vi "niWLAN - OPPO - 80211abgnIQMeasurementsSettings.vi"(0 "niwlan analysis session":T6, 1 "WLAN Measurement Settings":T1={"OFDM Advanced Controls(11ag)"={"OFDM Auto Compute Acquisition Length Enabled"=0, "OFDM Maximum Symbols Used"=0, "OFDM Time Tracking Enabled"=0, "OFDM Channel Tracking Enabled"=0, "OFDM Amplitude Tracking Enabled"=1, "OFDM CFO Estimation Method"=0, "OFDM Phase Tracking Method"=0, "OFDM Header Detection Enabled"=0, "OFDM MAC FCS Check Enabled"=0, "#Avg"=10, "#Iterations"=10}, "DSSS Demod Parameters"={"DSSS Auto Compute Acquisition Length Enabled"=0, "DSSS Equalization Enabled"=0, "DSSS Header Detection Enabled"=0, "DSSS MAC FCS Check Enabled"=0, "DSSS Measurement Start Location"=0, "DSSS Phase Tracking Method"=0, "DSSS Maximum Chips Used"=0, "DSSS Reference Pulse Shaping Filter"=0, "DSSS Reference Pulse Shaping Filter Coefficient"=0.0, "# Avg"=1024, "# Iterations"=1024, "DSSS Power Ramp Enabled"=0}, "OFDM Advanced Controls (11n)"={"OFDM Auto Compute Acquisition Length Enabled"=0, "OFDM Maximum Symbols Used"=0, "OFDM Time Tracking Enabled"=0, "OFDM Channel Tracking Enabled"=0, "OFDM Amplitude Tracking Enabled"=1, "OFDM CFO Estimation Method"=0, "OFDM Phase Tracking Method"=0, "OFDM Header Detection Enabled"=0, "OFDM MAC FCS Check Enabled"=0, "#Avg"=10, "#Iterations"=10}, "OFDM Advanced Controls(11ac)"={"OFDM Auto Compute Acquisition Length Enabled"=0, "OFDM Maximum Symbols Used"=0, "OFDM Time Tracking Enabled"=1, "OFDM Channel Tracking Enabled"=0, "OFDM Amplitude Tracking Enabled"=0, "OFDM CFO Estimation Method"=0, "OFDM Phase Tracking Method"=0, "OFDM Header Detection Enabled"=0, "OFDM MAC FCS Check Enabled"=0, "#Avg"=10, "#Iterations"=10}} {"OFDM Advanced Controls(11ac)"."OFDM Phase Tracking Method" items=["Standard", "Instantaneous", "None", "Standard with Cubic Spline Fit"]; "OFDM Advanced Controls(11ac)"."OFDM CFO Estimation Method" items=["Preamble Only", "Preamble and Data"]; "OFDM Advanced Controls(11ac)"."OFDM Channel Tracking Enabled" items=["False", "True"]; "OFDM Advanced Controls(11ac)"."OFDM Amplitude Tracking Enabled" items=["False", "True"]; "OFDM Advanced Controls(11ac)"."OFDM Time Tracking Enabled" items=["True"=1, "False"=0]; "OFDM Advanced Controls(11ac)"."OFDM Auto Compute Acquisition Length Enabled" items=["False", "True"]; "OFDM Advanced Controls(11ac)"."OFDM MAC FCS Check Enabled" items=["False", "True"]; "OFDM Advanced Controls(11ac)"."OFDM Header Detection Enabled" items=["False", "True"]; "OFDM Advanced Controls (11n)"."OFDM Phase Tracking Method" items=["Standard", "Instantaneous", "None", "Standard with Cubic Spline Fit"]; "OFDM Advanced Controls (11n)"."OFDM CFO Estimation Method" items=["Preamble Only", "Preamble and Data"]; "OFDM Advanced Controls (11n)"."OFDM Channel Tracking Enabled" items=["False", "True"]; "OFDM Advanced Controls (11n)"."OFDM Amplitude Tracking Enabled" items=["False", "True"]; "OFDM Advanced Controls (11n)"."OFDM Time Tracking Enabled" items=["True"=1, "False"=0]; "OFDM Advanced Controls (11n)"."OFDM Auto Compute Acquisition Length Enabled" items=["False", "True"]; "OFDM Advanced Controls (11n)"."OFDM MAC FCS Check Enabled" items=["False", "True"]; "OFDM Advanced Controls (11n)"."OFDM Header Detection Enabled" items=["False", "True"]; "DSSS Demod Parameters"."DSSS Power Ramp Enabled" items=["False", "True"]; "DSSS Demod Parameters"."DSSS Auto Compute Acquisition Length Enabled" items=["False", "True"]; "DSSS Demod Parameters"."DSSS Phase Tracking Method" items=["Standard", "Instantaneous"]; "DSSS Demod Parameters"."DSSS Equalization Enabled" items=["False", "True"]; "DSSS Demod Parameters"."DSSS Reference Pulse Shaping Filter" items=["Rectangular", "Raised Cosine", "Root Raised Cosine", "Gaussian"]; "DSSS Demod Parameters"."DSSS MAC FCS Check Enabled" items=["False", "True"]; "DSSS Demod Parameters"."DSSS Header Detection Enabled" items=["False", "True"]; "OFDM Advanced Controls(11ag)"."OFDM Phase Tracking Method" items=["Standard", "Instantaneous", "None", "Standard with Cubic Spline Fit"]; "OFDM Advanced Controls(11ag)"."OFDM CFO Estimation Method" items=["Preamble Only", "Preamble and Data"]; "OFDM Advanced Controls(11ag)"."OFDM Channel Tracking Enabled" items=["False", "True"]; "OFDM Advanced Controls(11ag)"."OFDM Amplitude Tracking Enabled" items=["False", "True"]; "OFDM Advanced Controls(11ag)"."OFDM Time Tracking Enabled" items=["True"=1, "False"=0]; "OFDM Advanced Controls(11ag)"."OFDM Auto Compute Acquisition Length Enabled" items=["False", "True"]; "OFDM Advanced Controls(11ag)"."OFDM MAC FCS Check Enabled" items=["False", "True"]; "OFDM Advanced Controls(11ag)"."OFDM Header Detection Enabled" items=["False", "True"]}, 2 "Measurement Type":T4(ring), 5 "TV Parameters(DataType)":T5 {"Standard" items=["80211A/G/J/P OFDM", "80211B/G DSSS", "80211G DSSSOFDM", "80211N MIMOOFDM", "80211AC MIMOOFDM"]; "OFDM Data Rate (Mbps)" items=["6", "9", "12", "18", "24", "36", "48", "54"]; "80211n PLCP Frame Format" items=["Mixed Format", "Greenfield Format"]; "FEC Coding Type" items=["BCC", "LDPC"]; "DSSS Data Rate (Mbps)" items=["1", "2", "5.5 CCK", "5.5 PBCC", "11 CCK", "11 PBCC", "22", "33"]}, 7 "Set TV ?":bool, 9 "Acquisition Length (s)":dbl=0.002, 11 "error in":errorcluster, 13 "Cal Routine ?":bool) -> (4 "niWLAN session":T6, 15 "error out":errorcluster)   [LabVIEW 2012]
uses:
  <vilib>/RF Toolkits/WLAN/analysis/controls/wlanv1 Analysis Refnum.ctl
  TV/RW/Includes/WLAN - TV - RW - INC - TV_DataType_Cluster.ctl
  TV/RW/Includes/WLAN - TV - RW - INC - Tx_Measurement_Cluster.ctl
  TV/RW/Includes/WLAN - TV - RW - INC - TV_OFDM Demod.ctl
  TV/RW/Includes/WLAN - TV - RW - INC - TV_DSSS Demod.ctl
  <resource>/objmgr/niWLANAnalysis.rc
panel:
  # "Hardware Configuration"
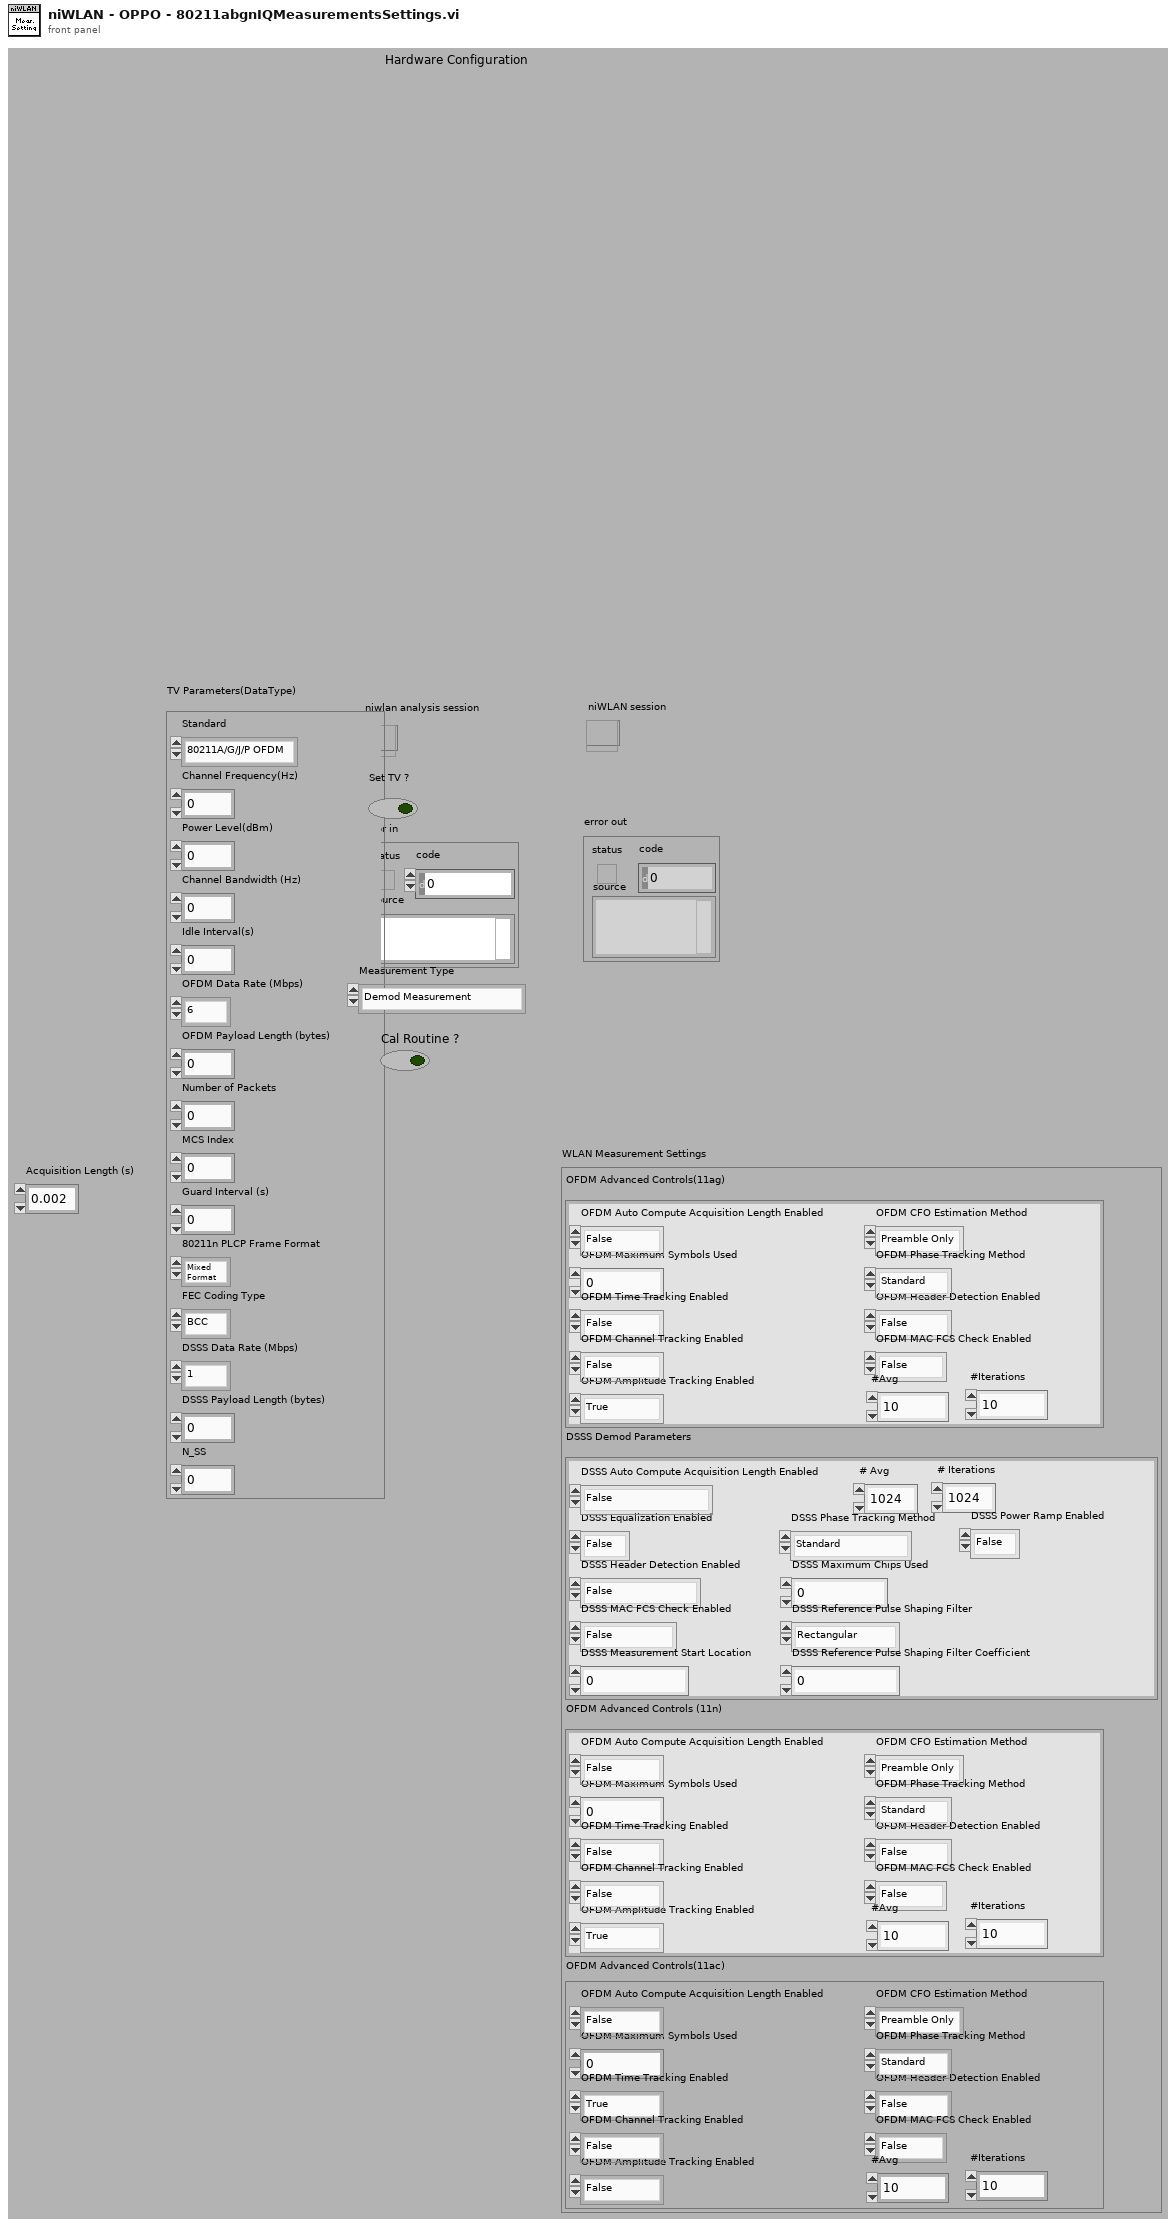
[diagram p1: front panel]
types:
  T1 = typedef "WLAN - TV - RW - INC - Tx_Measurement_Cluster.ctl" = cluster{"OFDM Advanced Controls(11ag)":T2, "DSSS Demod Parameters":T3, "OFDM Advanced Controls (11n)":T2, "OFDM Advanced Controls(11ac)":cluster{"OFDM Auto Compute Acquisition Length Enabled":i32, "OFDM Maximum Symbols Used":i32, "OFDM Time Tracking Enabled":i32, "OFDM Channel Tracking Enabled":i32, "OFDM Amplitude Tracking Enabled":i32, "OFDM CFO Estimation Method":i32, "OFDM Phase Tracking Method":i32, "OFDM Header Detection Enabled":i32, "OFDM MAC FCS Check Enabled":i32, "#Avg":i32, "#Iterations":i32}}
  T2 = typedef "WLAN - TV - RW - INC - TV_OFDM Demod.ctl" = cluster{"OFDM Auto Compute Acquisition Length Enabled":i32, "OFDM Maximum Symbols Used":i32, "OFDM Time Tracking Enabled":i32, "OFDM Channel Tracking Enabled":i32, "OFDM Amplitude Tracking Enabled":i32, "OFDM CFO Estimation Method":i32, "OFDM Phase Tracking Method":i32, "OFDM Header Detection Enabled":i32, "OFDM MAC FCS Check Enabled":i32, "#Avg":i32, "#Iterations":i32}
  T3 = typedef "WLAN - TV - RW - INC - TV_DSSS Demod.ctl" = cluster{"DSSS Auto Compute Acquisition Length Enabled":i32, "DSSS Equalization Enabled":i32, "DSSS Header Detection Enabled":i32, "DSSS MAC FCS Check Enabled":i32, "DSSS Measurement Start Location":i32, "DSSS Phase Tracking Method":i32, "DSSS Maximum Chips Used":i32, "DSSS Reference Pulse Shaping Filter":i32, "DSSS Reference Pulse Shaping Filter Coefficient":dbl, "# Avg":i32, "# Iterations":i32, "DSSS Power Ramp Enabled":i32}
  T4 = enum16{"Demod Measurement", "Spectrum Measurement"}
  T5 = typedef "WLAN - TV - RW - INC - TV_DataType_Cluster.ctl" = cluster{"Standard":i32, "Channel Frequency(Hz)":dbl, "Power Level(dBm)":dbl, "Channel Bandwidth (Hz)":dbl, "Idle Interval(s)":dbl, "OFDM Data Rate (Mbps)":i32, "OFDM Payload Length (bytes)":i32, "Number of Packets":i32, "MCS Index":i32, "Guard Interval (s)":dbl, "80211n PLCP Frame Format":i32, "FEC Coding Type":i32, "DSSS Data Rate (Mbps)":i32, "DSSS Payload Length (bytes)":i32, "N_SS":i32}
  T6 = typedef "wlanv1 Analysis Refnum.ctl" = refnum<k20>
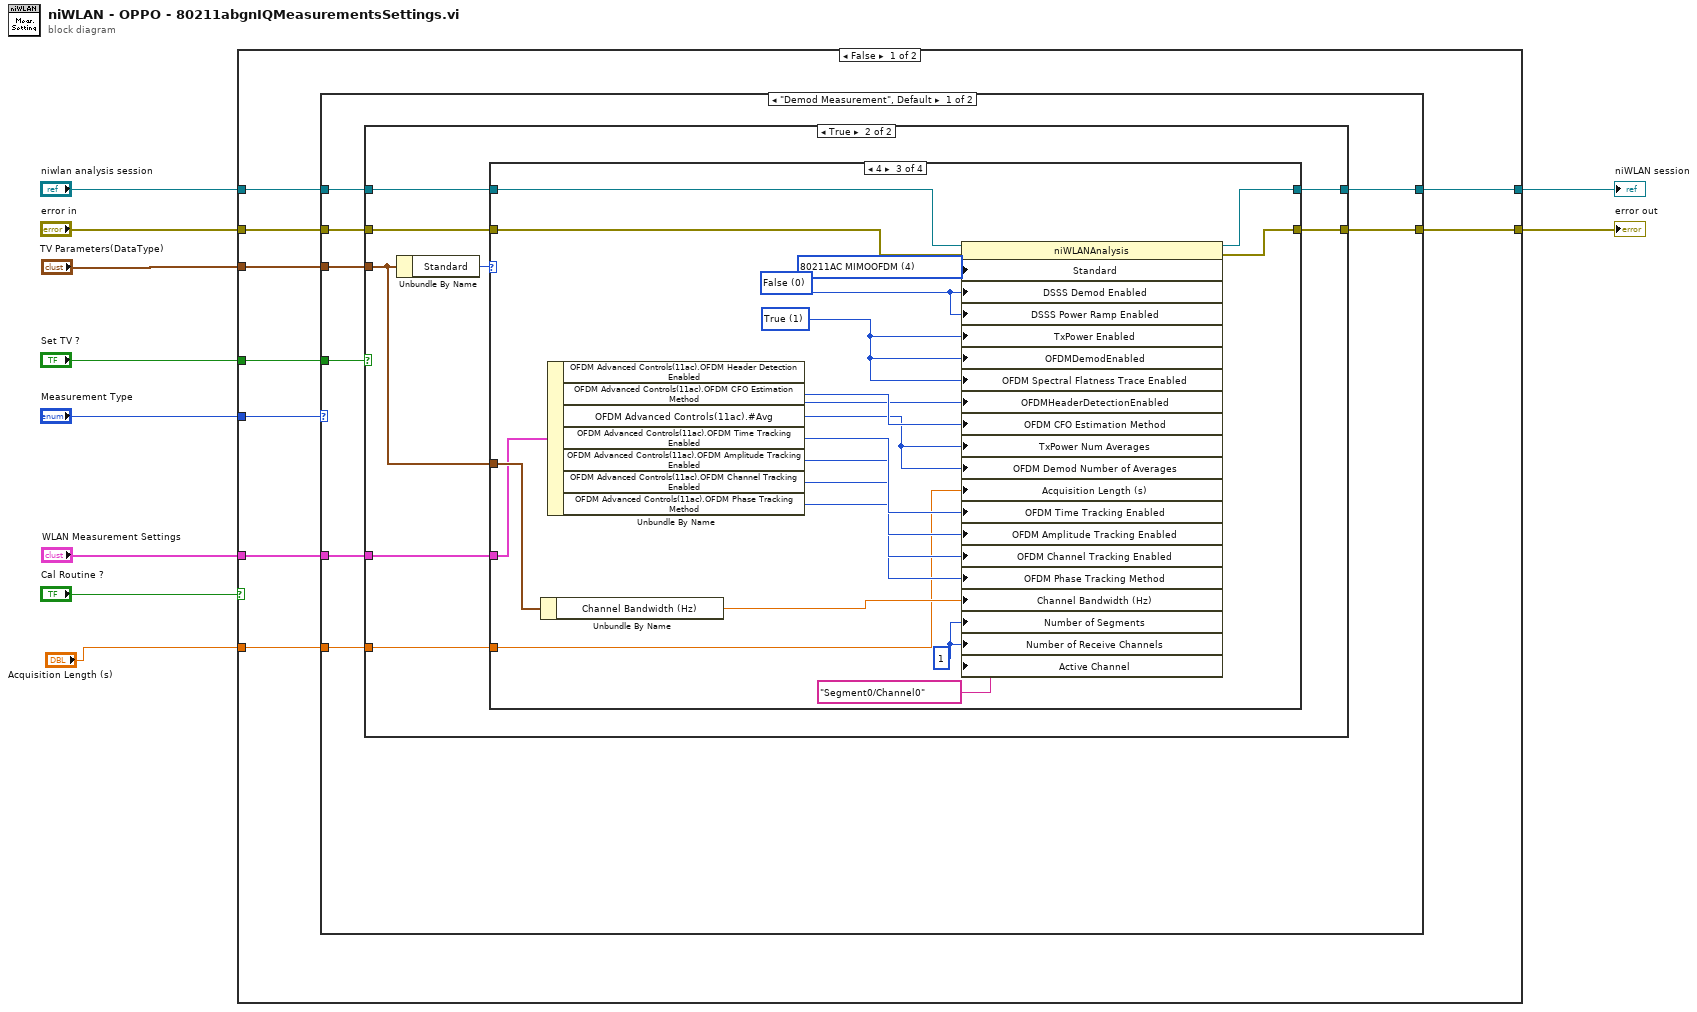
[diagram p0: block diagram]
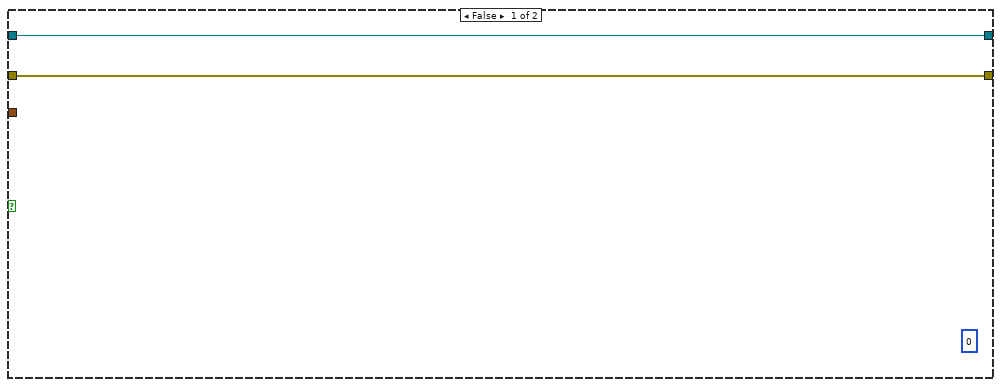
[diagram p2: hidden frame]
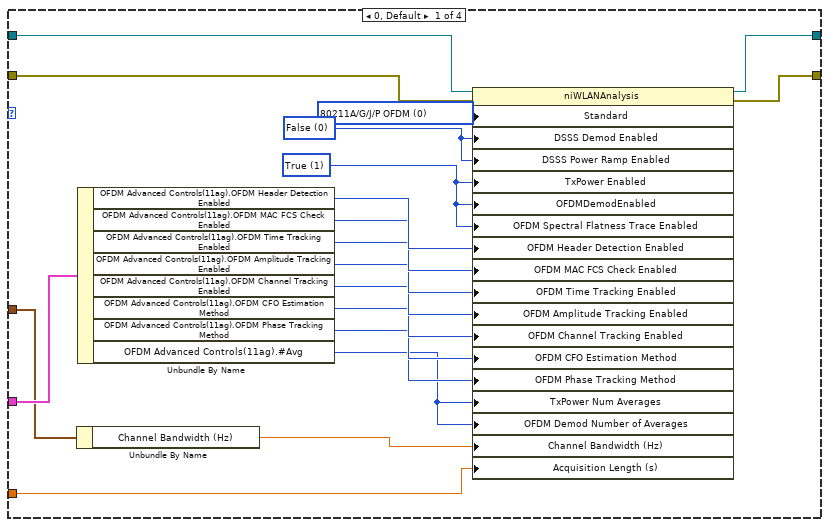
[diagram p3: hidden frame]
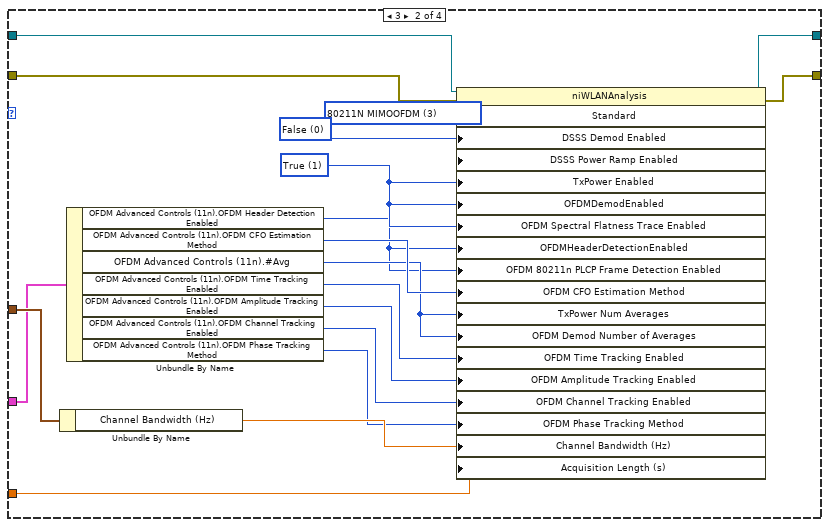
[diagram p4: hidden frame]
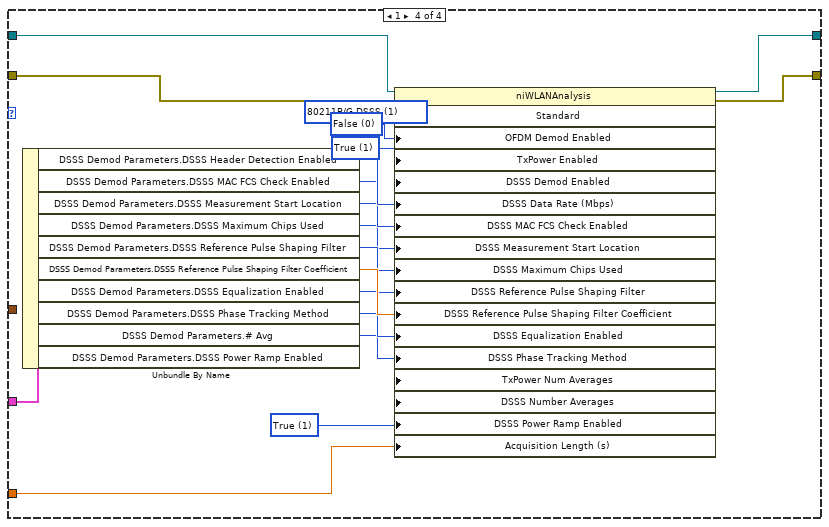
[diagram p5: hidden frame]
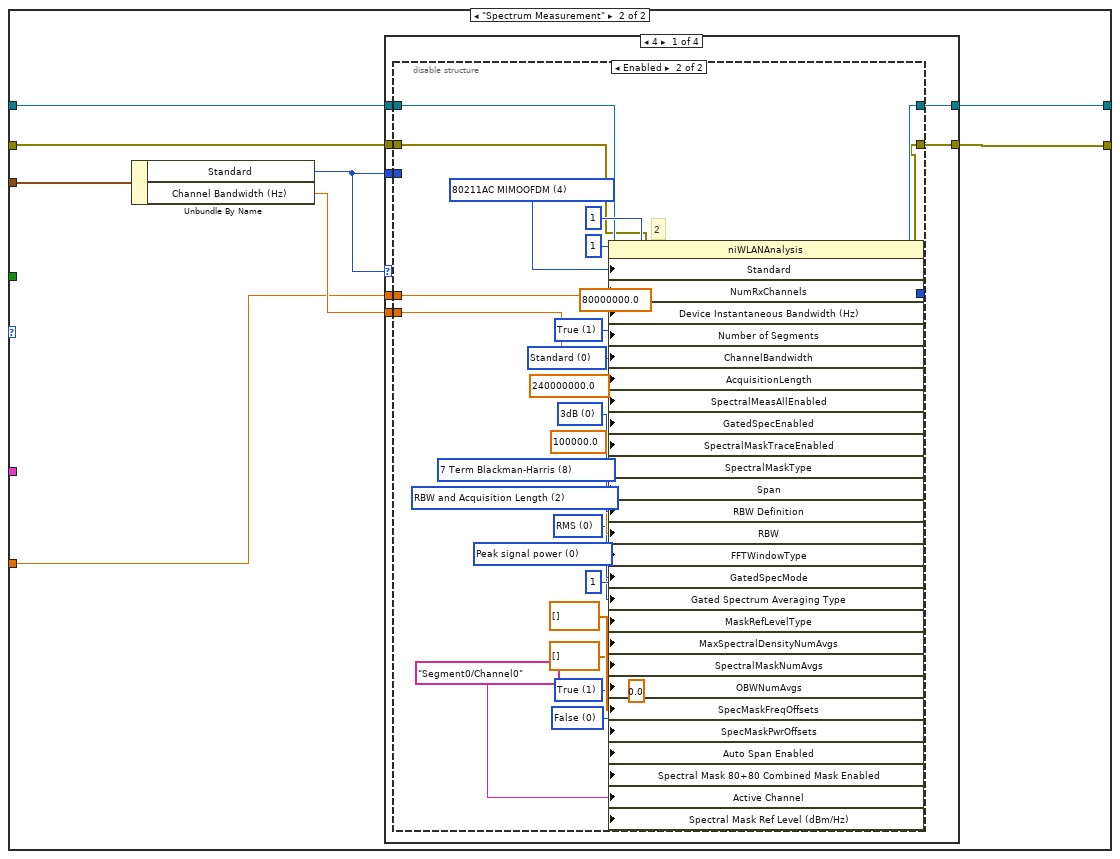
[diagram p6: hidden frame]
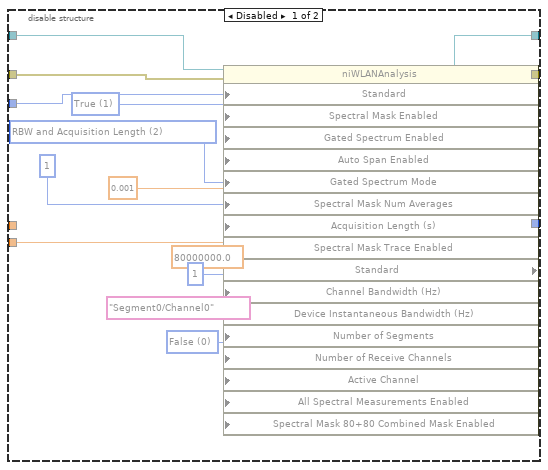
[diagram p7: hidden frame]
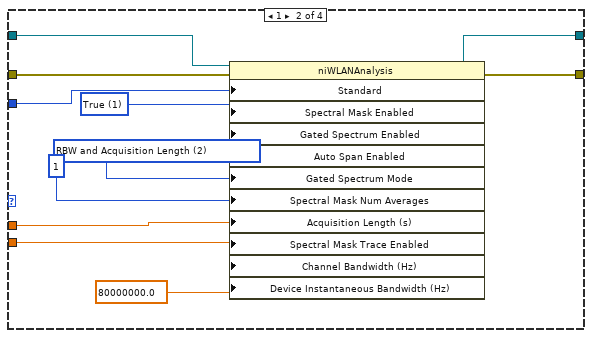
[diagram p8: hidden frame]
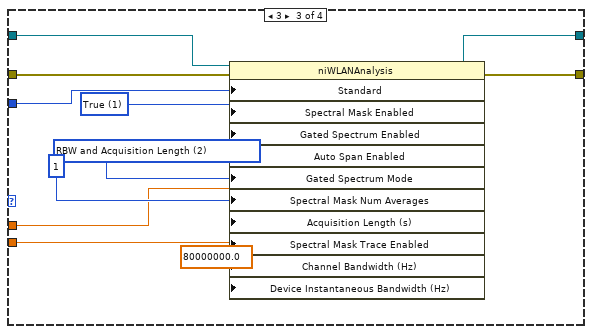
[diagram p9: hidden frame]
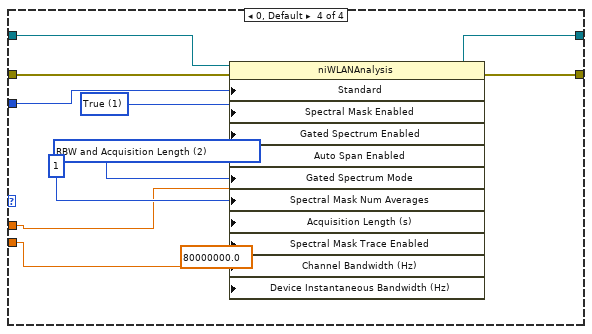
[diagram p10: hidden frame]
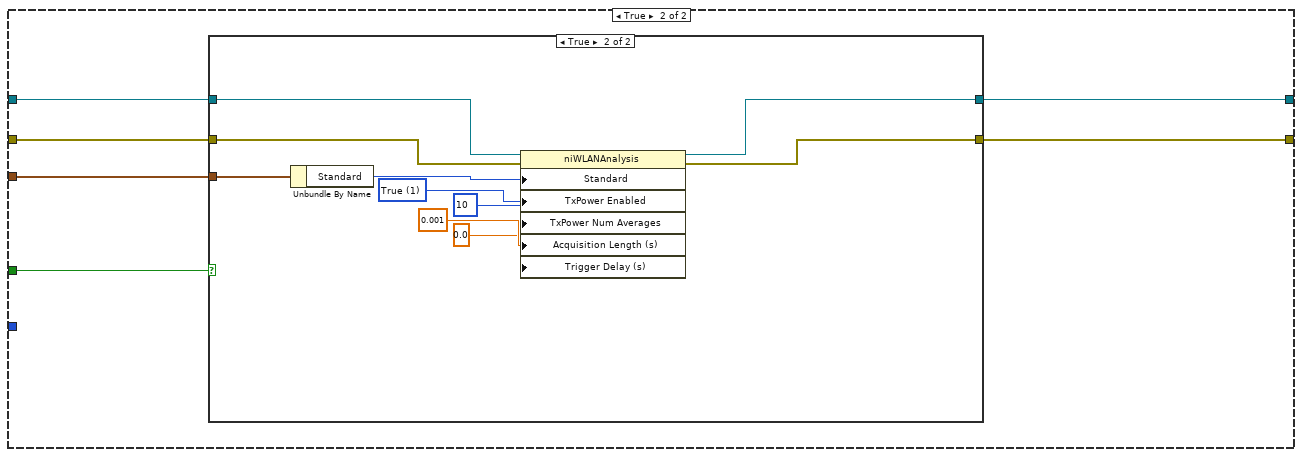
[diagram p11: hidden frame]
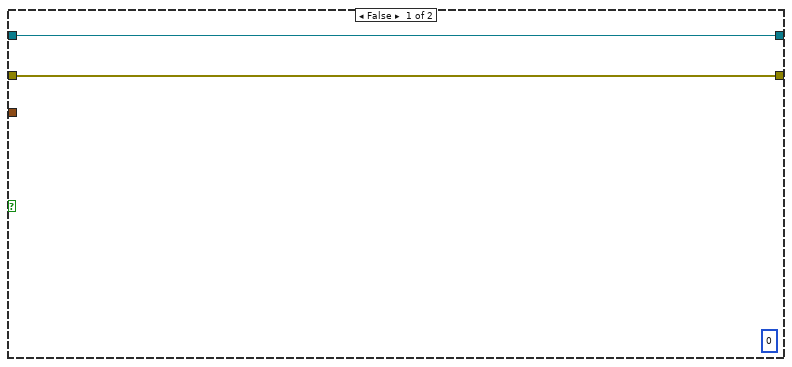
[diagram p12: hidden frame]
diagram:
  n1 = case shown="False" "Cal Routine ?" {
    tunnel: "niwlan analysis session" -> [w19 w208]
    tunnel: "error in" -> [w18 w207]
    tunnel: [w17 w206] -> w8
    tunnel: [w16 w205] -> w7
    tunnel: "TV Parameters(DataType)" -> [w15 w204]
    tunnel: "Set TV ?" -> [w14 w203]
    tunnel: "Measurement Type" -> [w13 _]
    tunnel: "WLAN Measurement Settings" -> [w12 _]
    tunnel: "Acquisition Length (s)" -> [w11 _]
    frame False {
      n2 = case shown="\"Demod Measurement\", Default" w13 {
        tunnel: w19 -> [w27 w121]
        tunnel: w18 -> [w26 w120]
        tunnel: [w25 w118] -> w17
        tunnel: [w24 w117] -> w16
        tunnel: w15 -> [w23 w119]
        tunnel: w14 -> [w22 _]
        tunnel: w12 -> [w21 _]
        tunnel: w11 -> [w20 w114]
        frame "Demod Measurement", Default {
          n3 = case shown="True" w22 {
            tunnel: w27 -> [w29 w37]
            tunnel: w26 -> [w28 w36]
            tunnel: [w29 w35] -> w25
            tunnel: [w28 w34] -> w24
            tunnel: w23 -> [_ w32]
            tunnel: w21 -> [_ w31]
            tunnel: w20 -> [_ w30]
            frame False {
              (unwired) 0 ("Standard")
            }
            frame True {
              n4 = Unbundle By Name(w32) -> ("Standard"=w33:i32)
              n5 = case shown="4" w33 {
                tunnel: w37 -> [w56 w74 w94 w113]
                tunnel: w36 -> [w55 w73 w93 w112]
                tunnel: [w54 w72 w92 w111] -> w35
                tunnel: [w53 w71 w91 w110] -> w34
                tunnel: w32 -> [w42 w70 w90 _]
                tunnel: w31 -> [w52 w68 w88 w107]
                tunnel: w30 -> [w38 w57 w76 w96]
                frame 0, Default {
                  w39 = 0 items=["80211A/G/J/P OFDM", "80211B/G DSSS", "80211G DSSSOFDM", "80211N MIMOOFDM", "80211AC MIMOOFDM"] ("Standard")
                  w40 = 0 items=["False", "True"] ("DSSS Demod Enabled")
                  w51 = 1 items=["False", "True"] ("OFDMDemodEnabled")
                  n6 = Unbundle By Name(w42) -> ("Channel Bandwidth (Hz)"=w41:dbl)
                  n7 = Unbundle By Name(w52) -> ("OFDM Advanced Controls(11ag).OFDM Header Detection Enabled"=w50:i32, "OFDM Advanced Controls(11ag).OFDM MAC FCS Check Enabled"=w49:i32, "OFDM Advanced Controls(11ag).OFDM Time Tracking Enabled"=w48:i32, "OFDM Advanced Controls(11ag).OFDM Amplitude Tracking Enabled"=w47:i32, "OFDM Advanced Controls(11ag).OFDM Channel Tracking Enabled"=w46:i32, "OFDM Advanced Controls(11ag).OFDM CFO Estimation Method"=w45:i32, "OFDM Advanced Controls(11ag).OFDM Phase Tracking Method"=w44:i32, "OFDM Advanced Controls(11ag).#Avg"=w43:i32)
                  n8 = property class="niWLANAnalysis"(reference=w56, error in=w55, "Standard"=w39, "DSSS Demod Enabled"=w40, "DSSS Power Ramp Enabled"=w40, "TxPower Enabled"=w51, "OFDMDemodEnabled"=w51, "OFDM Spectral Flatness Trace Enabled"=w51, "OFDM Header Detection Enabled"=w50, "OFDM MAC FCS Check Enabled"=w49, "OFDM Time Tracking Enabled"=w48, "OFDM Amplitude Tracking Enabled"=w47, "OFDM Channel Tracking Enabled"=w46, "OFDM CFO Estimation Method"=w45, "OFDM Phase Tracking Method"=w44, "TxPower Num Averages"=w43, "OFDM Demod Number of Averages"=w43, "Channel Bandwidth (Hz)"=w41, "Acquisition Length (s)"=w38) -> (reference out=w54:T6, error out=w53:errorcluster)
                }
                frame 3 {
                  w58 = 3 items=["80211A/G/J/P OFDM", "80211B/G DSSS", "80211G DSSSOFDM", "80211N MIMOOFDM", "80211AC MIMOOFDM"] ("Standard")
                  w59 = 0 items=["False", "True"] ("OFDMDemodEnabled")
                  w62 = 1 items=["False", "True"] ("OFDMDemodEnabled")
                  n9 = Unbundle By Name(w70) -> ("Channel Bandwidth (Hz)"=w69:dbl)
                  n10 = Unbundle By Name(w68) -> ("OFDM Advanced Controls (11n).OFDM Header Detection Enabled"=w60:i32, "OFDM Advanced Controls (11n).OFDM CFO Estimation Method"=w67:i32, "OFDM Advanced Controls (11n).#Avg"=w61:i32, "OFDM Advanced Controls (11n).OFDM Time Tracking Enabled"=w66:i32, "OFDM Advanced Controls (11n).OFDM Amplitude Tracking Enabled"=w65:i32, "OFDM Advanced Controls (11n).OFDM Channel Tracking Enabled"=w64:i32, "OFDM Advanced Controls (11n).OFDM Phase Tracking Method"=w63:i32)
                  n11 = property class="niWLANAnalysis"(reference=w74, error in=w73, "Standard"=w58, "DSSS Demod Enabled"=w59, "DSSS Power Ramp Enabled"=w59, "TxPower Enabled"=w62, "OFDMDemodEnabled"=w62, "OFDM Spectral Flatness Trace Enabled"=w62, "OFDMHeaderDetectionEnabled"=w60, "OFDM 80211n PLCP Frame Detection Enabled"=w60, "OFDM CFO Estimation Method"=w67, "TxPower Num Averages"=w61, "OFDM Demod Number of Averages"=w61, "OFDM Time Tracking Enabled"=w66, "OFDM Amplitude Tracking Enabled"=w65, "OFDM Channel Tracking Enabled"=w64, "OFDM Phase Tracking Method"=w63, "Channel Bandwidth (Hz)"=w69, "Acquisition Length (s)"=w57) -> (reference out=w72:T6, error out=w71:errorcluster)
                }
                frame 4 {
                  w77 = 4 items=["80211A/G/J/P OFDM", "80211B/G DSSS", "80211G DSSSOFDM", "80211N MIMOOFDM", "80211AC MIMOOFDM"] ("Standard")
                  w79 = 1 ("Number of Segments")
                  w80 = 0 items=["False", "True"] ("OFDMDemodEnabled")
                  w82 = 1 items=["False", "True"] ("OFDMDemodEnabled")
                  n12 = Unbundle By Name(w90) -> ("Channel Bandwidth (Hz)"=w89:dbl)
                  n13 = Unbundle By Name(w88) -> ("OFDM Advanced Controls(11ac).OFDM Header Detection Enabled"=w75:i32, "OFDM Advanced Controls(11ac).OFDM CFO Estimation Method"=w87:i32, "OFDM Advanced Controls(11ac).#Avg"=w81:i32, "OFDM Advanced Controls(11ac).OFDM Time Tracking Enabled"=w86:i32, "OFDM Advanced Controls(11ac).OFDM Amplitude Tracking Enabled"=w85:i32, "OFDM Advanced Controls(11ac).OFDM Channel Tracking Enabled"=w84:i32, "OFDM Advanced Controls(11ac).OFDM Phase Tracking Method"=w83:i32)
                  n14 = property class="niWLANAnalysis"(reference=w94, error in=w93, "Standard"=w77, "DSSS Demod Enabled"=w80, "DSSS Power Ramp Enabled"=w80, "TxPower Enabled"=w82, "OFDMDemodEnabled"=w82, "OFDM Spectral Flatness Trace Enabled"=w82, "OFDMHeaderDetectionEnabled"=w75, "OFDM CFO Estimation Method"=w87, "TxPower Num Averages"=w81, "OFDM Demod Number of Averages"=w81, "Acquisition Length (s)"=w76, "OFDM Time Tracking Enabled"=w86, "OFDM Amplitude Tracking Enabled"=w85, "OFDM Channel Tracking Enabled"=w84, "OFDM Phase Tracking Method"=w83, "Channel Bandwidth (Hz)"=w89, "Number of Segments"=w79, "Number of Receive Channels"=w79, "Active Channel"="Segment0/Channel0") -> (reference out=w92:T6, error out=w91:errorcluster)
                }
                frame 1 {
                  w95 = 1 items=["False", "True"] ("DSSS Power Ramp Enabled")
                  w97 = 1 items=["80211A/G/J/P OFDM", "80211B/G DSSS", "80211G DSSSOFDM", "80211N MIMOOFDM", "80211AC MIMOOFDM"] ("Standard")
                  w108 = 0 items=["False", "True"] ("OFDM Demod Enabled")
                  w109 = 1 items=["False", "True"] ("OFDMDemodEnabled")
                  n15 = Unbundle By Name(w107) -> ("DSSS Demod Parameters.DSSS Header Detection Enabled"=w104:i32, "DSSS Demod Parameters.DSSS MAC FCS Check Enabled"=w103:i32, "DSSS Demod Parameters.DSSS Measurement Start Location"=w102:i32, "DSSS Demod Parameters.DSSS Maximum Chips Used"=w101:i32, "DSSS Demod Parameters.DSSS Reference Pulse Shaping Filter"=w105:i32, "DSSS Demod Parameters.DSSS Reference Pulse Shaping Filter Coefficient"=w106:dbl, "DSSS Demod Parameters.DSSS Equalization Enabled"=w100:i32, "DSSS Demod Parameters.DSSS Phase Tracking Method"=w99:i32, "DSSS Demod Parameters.# Avg"=w98:i32)  [unwired: 1 out]
                  n16 = property class="niWLANAnalysis"(reference=w113, error in=w112, "Standard"=w97, "OFDM Demod Enabled"=w108, "TxPower Enabled"=w109, "DSSS Demod Enabled"=w109, "DSSS Data Rate (Mbps)"=w104, "DSSS MAC FCS Check Enabled"=w103, "DSSS Measurement Start Location"=w102, "DSSS Maximum Chips Used"=w101, "DSSS Reference Pulse Shaping Filter"=w105, "DSSS Reference Pulse Shaping Filter Coefficient"=w106, "DSSS Equalization Enabled"=w100, "DSSS Phase Tracking Method"=w99, "TxPower Num Averages"=w98, "DSSS Number Averages"=w98, "DSSS Power Ramp Enabled"=w95, "Acquisition Length (s)"=w96) -> (reference out=w111:T6, error out=w110:errorcluster)
                }
              }
            }
          }
        }
        frame "Spectrum Measurement" {
          n17 = Unbundle By Name(w119) -> ("Standard"=w115:i32, "Channel Bandwidth (Hz)"=w116:dbl)
          n18 = case shown="4" w115 {
            tunnel: w121 -> [w128 w180 w191 w202]
            tunnel: w120 -> [w127 w179 w190 w201]
            tunnel: [w126 w178 w189 w200] -> w118
            tunnel: [w125 w177 w188 w199] -> w117
            tunnel: w115 -> [w124 w176 w187 w198]
            tunnel: w116 -> [w123 w172 w183 w194]
            tunnel: w114 -> [w122 w170 w181 w192]
            frame 4 {
              n19 = disable-structure shown="Enabled" {
                disable-tunnel: w128 -> [w143 w153]
                disable-tunnel: w127 -> [w142 w150]
                disable-tunnel: [w141 w152] -> w126
                disable-tunnel: [w140 w151] -> w125
                disable-tunnel: [w139 _] -> _
                disable-tunnel: w124 -> [w138 _]
                disable-tunnel: w123 -> [w134 w149]
                disable-tunnel: w122 -> [_ w144]
                frame Disabled {
                  w129 = 0 items=["False", "True"] ("Spectral Mask 80+80 Combined Mask Enabled")
                  w132 = 1 ("Number of Segments")
                  w136 = 2 items=["RBW", "Acquisition Length", "RBW and Acquisition Length"] ("Gated Spectrum Mode")
                  w130 = 1 items=["False", "True"] ("OFDMDemodEnabled")
                  n20 = property class="niWLANAnalysis"(reference=w143, error in=w142, "Standard"=w138, "Spectral Mask Enabled"=w130, "Gated Spectrum Enabled"=w130, "Auto Span Enabled"=w130, "Gated Spectrum Mode"=w136, "Spectral Mask Num Averages"=1 ("Averages"), "Acquisition Length (s)"=0.001, "Spectral Mask Trace Enabled"=w130, "Channel Bandwidth (Hz)"=w134, "Device Instantaneous Bandwidth (Hz)"=80000000.0, "Number of Segments"=w132, "Number of Receive Channels"=w132, "Active Channel"="Segment0/Channel0", "All Spectral Measurements Enabled"=w130, "Spectral Mask 80+80 Combined Mask Enabled"=w129) -> (reference out=w141:T6, error out=w140:errorcluster, "Standard"=w139:i32)
                }
                frame Enabled {
                  w158 = 0 items=["True"=1, "False"=0] ("Combine 80+80 Mask Enabled")
                  w159 = 1 items=["False", "True"] ("Auto Span Enabled")
                  w168 = 1 ("Number of Averages")
                  w161 = 0 items=["Peak signal power", "User defined"] ("Mask Reference Level Type")
                  w154 = 0 items=["RMS", "Log"] ("Gated Spectrum Averaging Type")
                  w164 = 2 items=["RBW", "Acquisition Length", "RBW and Acquisition Length"] ("Gated Spectrum Mode")
                  w165 = 8 items=["Uniform", "Hanning", "Hamming", "Blackman-Harris", "Exact Blackman", "Blackman", "Flat Top", "4 Term Blackman-Harris", "7 Term Blackman-Harris", "Low Side Lobe"] ("FFT Window Type")
                  w167 = 0 items=["3dB", "6dB", "ENBW", "bin width"] ("RBW Definition")
                  w155 = 0 items=["Standard", "User defined", "Standard at 5GHz"] ("Spectral Mask Type")
                  w146 = 4 items=["80211A/G/J/P OFDM", "80211B/G DSSS", "80211G DSSSOFDM", "80211N MIMOOFDM", "80211AC MIMOOFDM"] ("Standard")
                  w169 = 1 items=["False", "True"] ("SpectralMeasAllEnabled")
                  # "2"
                  n21 = property class="niWLANAnalysis"(reference=w153, error in=w150, "Standard"=w146, "NumRxChannels"=1 ("Number of Receive Channel"), "Device Instantaneous Bandwidth (Hz)"=80000000.0, "Number of Segments"=1 ("No. of Segments"), "ChannelBandwidth"=w149, "AcquisitionLength"=w144, "SpectralMeasAllEnabled"=w169, "GatedSpecEnabled"=w169, "SpectralMaskTraceEnabled"=w169, "SpectralMaskType"=w155, "Span"=240000000.0 ("Span (Hz)"), "RBW Definition"=w167, "RBW"=100000.0 ("RBW (Hz)"), "FFTWindowType"=w165, "GatedSpecMode"=w164, "Gated Spectrum Averaging Type"=w154, "MaskRefLevelType"=w161, "MaxSpectralDensityNumAvgs"=w168, "SpectralMaskNumAvgs"=w168, "OBWNumAvgs"=w168, "SpecMaskFreqOffsets"=dbl[] [] ("Spectral Mask Frequency Offset (Hz)"), "SpecMaskPwrOffsets"=dbl[] [] ("Spectral Mask Power Offset(dB)"), "Auto Span Enabled"=w159, "Spectral Mask 80+80 Combined Mask Enabled"=w158, "Active Channel"="Segment0/Channel0", "Spectral Mask Ref Level (dBm/Hz)"=0.0) -> (reference out=w152:T6, error out=w151:errorcluster)
                }
              }
            }
            frame 1 {
              w175 = 2 items=["RBW", "Acquisition Length", "RBW and Acquisition Length"] ("Gated Spectrum Mode")
              w173 = 1 items=["False", "True"] ("OFDMDemodEnabled")
              n22 = property class="niWLANAnalysis"(reference=w180, error in=w179, "Standard"=w176, "Spectral Mask Enabled"=w173, "Gated Spectrum Enabled"=w173, "Auto Span Enabled"=w173, "Gated Spectrum Mode"=w175, "Spectral Mask Num Averages"=1 ("Averages"), "Acquisition Length (s)"=w170, "Spectral Mask Trace Enabled"=w173, "Channel Bandwidth (Hz)"=w172, "Device Instantaneous Bandwidth (Hz)"=80000000.0) -> (reference out=w178:T6, error out=w177:errorcluster)
            }
            frame 3 {
              w186 = 2 items=["RBW", "Acquisition Length", "RBW and Acquisition Length"] ("Gated Spectrum Mode")
              w184 = 1 items=["False", "True"] ("OFDMDemodEnabled")
              n23 = property class="niWLANAnalysis"(reference=w191, error in=w190, "Standard"=w187, "Spectral Mask Enabled"=w184, "Gated Spectrum Enabled"=w184, "Auto Span Enabled"=w184, "Gated Spectrum Mode"=w186, "Spectral Mask Num Averages"=1 ("Averages"), "Acquisition Length (s)"=w181, "Spectral Mask Trace Enabled"=w184, "Channel Bandwidth (Hz)"=w183, "Device Instantaneous Bandwidth (Hz)"=80000000.0) -> (reference out=w189:T6, error out=w188:errorcluster)
            }
            frame 0, Default {
              w197 = 2 items=["RBW", "Acquisition Length", "RBW and Acquisition Length"] ("Gated Spectrum Mode")
              w195 = 1 items=["False", "True"] ("OFDMDemodEnabled")
              n24 = property class="niWLANAnalysis"(reference=w202, error in=w201, "Standard"=w198, "Spectral Mask Enabled"=w195, "Gated Spectrum Enabled"=w195, "Auto Span Enabled"=w195, "Gated Spectrum Mode"=w197, "Spectral Mask Num Averages"=1 ("Averages"), "Acquisition Length (s)"=w192, "Spectral Mask Trace Enabled"=w195, "Channel Bandwidth (Hz)"=w194, "Device Instantaneous Bandwidth (Hz)"=80000000.0) -> (reference out=w200:T6, error out=w199:errorcluster)
            }
          }
        }
      }
    }
    frame True {
      n25 = case shown="True" w203 {
        tunnel: w208 -> [w210 w220]
        tunnel: w207 -> [w209 w219]
        tunnel: [w210 w218] -> w206
        tunnel: [w209 w217] -> w205
        tunnel: w204 -> [_ w215]
        frame False {
          (unwired) 0 ("Standard")
        }
        frame True {
          w212 = 1 items=["False", "True"] ("OFDMDemodEnabled")
          n26 = Unbundle By Name(w215) -> ("Standard"=w216:i32)
          n27 = property class="niWLANAnalysis"(reference=w220, error in=w219, "Standard"=w216, "TxPower Enabled"=w212, "TxPower Num Averages"=10, "Acquisition Length (s)"=0.001, "Trigger Delay (s)"=0.0 ("Trigger Delay (sec)")) -> (reference out=w218:T6, error out=w217:errorcluster)
        }
      }
    }
  }
  "error out" <- w7
  "niWLAN session" <- w8
